vi "Scripting_UpdateBundle.vi"(8 "error in (no error)":errorcluster, 9 "Boolean":bool, 10 "PropertyName":string, 11 "VI in":refnum<vi>) -> (0 "error out":errorcluster)   [LabVIEW 2014]
panel:
  out "Full Element Names[]":cluster{string[]}[](array[cluster])
  out "Element Names[]":string[](array[string])
  out "Available Elements[]":string[](array[string])
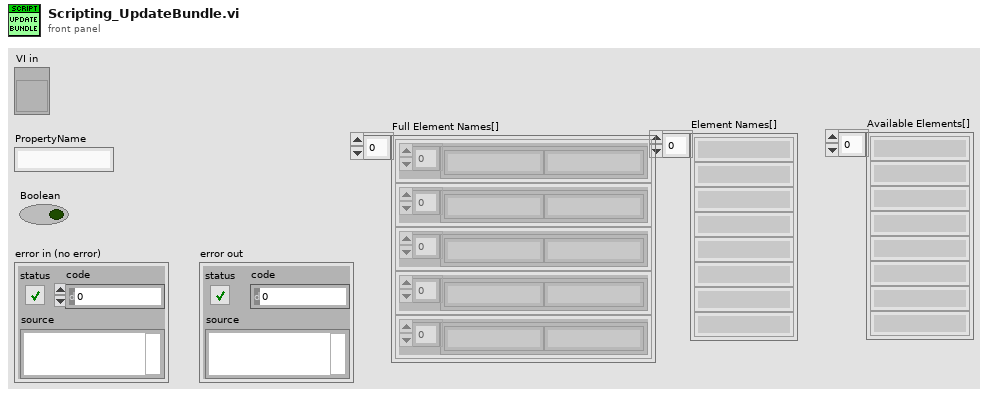
[diagram p1: front panel]
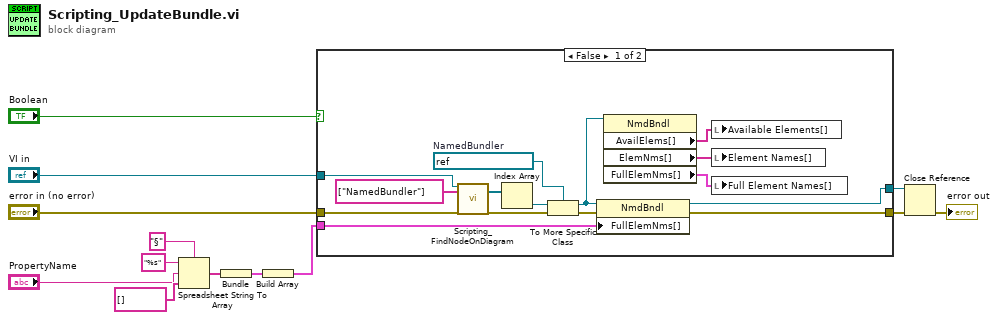
[diagram p0: block diagram]
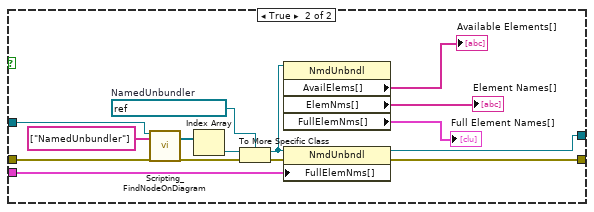
[diagram p2: hidden frame]
diagram:
  n1 = Spreadsheet String To Array(delimiter (Tab)="§" ("search string"), format string="%s", spreadsheet string="PropertyName", array type (2D Dbl)=string[] [] ("appended array")) -> (array=w10:string[])
  n2 = Bundle("appended array"=w10) -> (w6:cluster{"appended array":string[]})  [unwired: 1 in]
  n3 = Build Array(w6) -> (w7:cluster{"appended array":string[]}[])
  n4 = case shown="False" "Boolean" {
    tunnel: "error in (no error)" -> [w23 w41]
    tunnel: "VI in" -> [w22 w38]
    tunnel: w7 -> [w18 w36]
    tunnel: [w20 w34] -> w8
    tunnel: [w19 w33] -> w9
    frame False {
      w26 = refnum<vi> refnum  # NamedBundler
      n5 = call <resource>:"Scripting_FindNodeOnDiagram.vi"("ViRef(Ignored If Not Wired)"=w22, "NodeTypesToSearchFor"=string[] ["NamedBundler"], "error in (no error)"=w23) -> ("Nodes"=w24:refnum<vi>[], "error out"=w28:errorcluster)  [unwired: 15 in]
      n6 = Index Array(array=w24) -> (element=w27:refnum<vi>)  [unwired: 1 in]
      n7 = To More Specific Class(target class=w26, reference=w27, error in=w28) -> (specific class reference=w17:refnum<vi>, error out=w21:errorcluster)
      n8 = property class="NmdBndl"(reference=w17, error in=w21, "FullElemNms[]"=w18) -> (reference out=w19:refnum<vi>, error out=w20:errorcluster)
      n9 = property class="NmdBndl"(reference=w17) -> ("AvailElems[]"=w15:string[], "ElemNms[]"=w14:string[], "FullElemNms[]"=w16:cluster{string[]}[])  [unwired: 1 in, 2 out]
      n10 = local write "Available Elements[]"(w15) -> ()
      n11 = local write "Element Names[]"(w14) -> ()
      n12 = local write "Full Element Names[]"(w16) -> ()
    }
    frame True {
      w35 = refnum<vi> refnum  # NamedUnbundler
      n13 = call <resource>:"Scripting_FindNodeOnDiagram.vi"("ViRef(Ignored If Not Wired)"=w38, "NodeTypesToSearchFor"=string[] ["NamedUnbundler"], "error in (no error)"=w41) -> ("Nodes"=w42:refnum<vi>[], "error out"=w40:errorcluster)  [unwired: 15 in]
      n14 = Index Array(array=w42) -> (element=w39:refnum<vi>)  [unwired: 1 in]
      n15 = To More Specific Class(target class=w35, reference=w39, error in=w40) -> (specific class reference=w32:refnum<vi>, error out=w37:errorcluster)
      n16 = property class="NmdUnbndl"(reference=w32) -> ("AvailElems[]"=→"Available Elements[]":string[], "ElemNms[]"=→"Element Names[]":string[], "FullElemNms[]"=→"Full Element Names[]":cluster{string[]}[])  [unwired: 1 in, 2 out]
      n17 = property class="NmdUnbndl"(reference=w32, error in=w37, "FullElemNms[]"=w36) -> (reference out=w33:refnum<vi>, error out=w34:errorcluster)
    }
  }
  n18 = Close Reference(reference=w9, error in (no error)=w8) -> (error out=→"error out":errorcluster)
